vi "Build Launch Nested Views Msg.vi"(8 "error in (no error)":errorcluster, 10 "View Labels":string[](array[string]), 11 "Nested Views":refnum<class "IViewable.lvclass">[](array[class])) -> (0 "error out":errorcluster, 3 "Launch Nested Views Msg out":refnum<class "Launch Nested Views Msg.lvclass">)   [LabVIEW 2015, in "IViewManager.lvlib" / "Launch Nested Views Msg.lvclass"]
uses:
  Launch Nested Views Msg.lvclass
  IViewable/IViewable/IViewable.lvclass
  Launch Nested Views Msg.lvclass/Launch Nested Views Msg.ctl
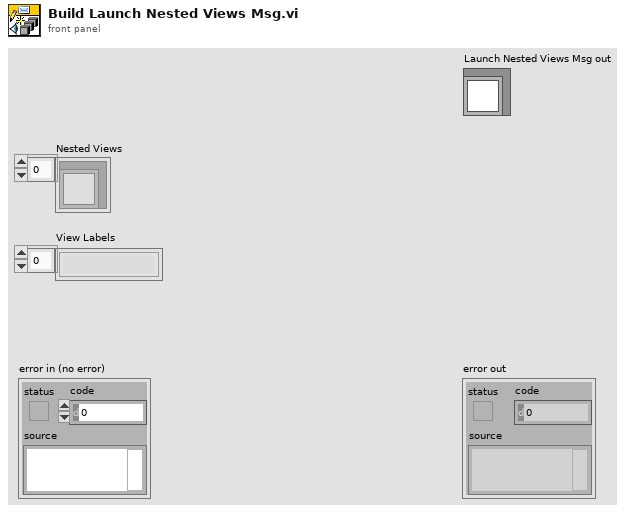
[diagram p1: front panel]
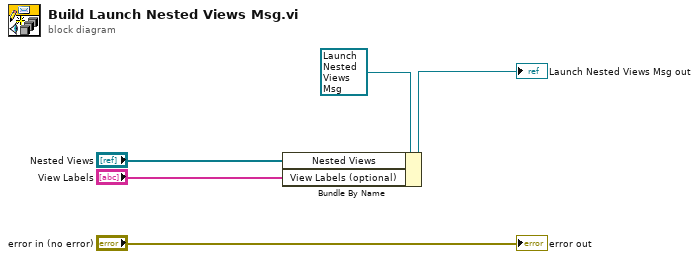
[diagram p0: block diagram]
diagram:
  n1 = Bundle By Name(cluster=refnum<class "Launch Nested Views Msg.lvclass"> refnum ("Launch Nested Views Msg in"), "Nested Views"="Nested Views", "View Labels (optional)"="View Labels") -> (→"Launch Nested Views Msg out":refnum<class "Launch Nested Views Msg.lvclass">)
  "error out" <- "error in (no error)"
